vi "Perdite da a vuoto.vi"(0 "Acquisizioni vuoto":T3, 1 "Acqisizioni termica":T2) -> (15 "Perdite da prova a vuoto":T1)   [LabVIEW 2019]
uses:
  <vilib>/Analysis/NI_AALPro.lvlib
panel:
  out "XY Graph":cluster{dbl[], dbl[]}[](graph)
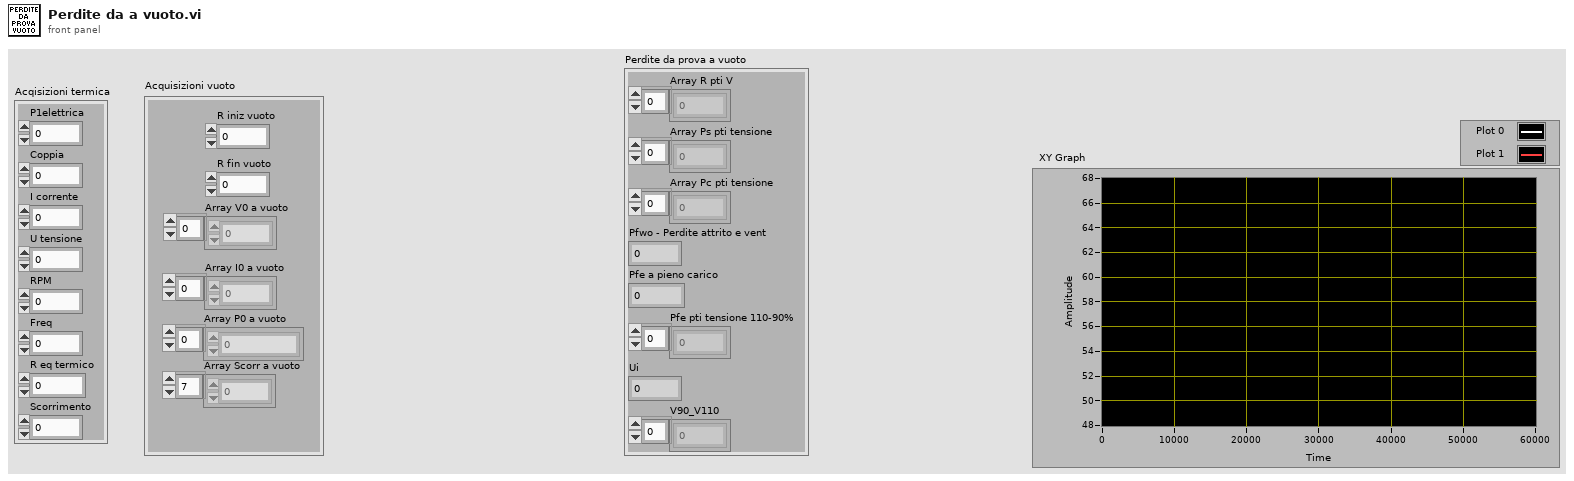
[diagram p1: front panel]
types:
  T1 = cluster{"Array R pti V":dbl[], "Array Ps pti tensione":dbl[], "Array Pc pti tensione":dbl[], "Pfwo - Perdite attrito e vent":dbl, "Pfe a pieno carico":dbl, "Pfe pti tensione 110-90% ":dbl[], "Ui":dbl, "V90_V110":dbl[]}
  T2 = cluster{"P1elettrica":dbl, "Coppia":dbl, "I corrente":dbl, "U tensione":dbl, "RPM":dbl, "Freq":dbl, "R eq termico":dbl, "Scorrimento":dbl}
  T3 = cluster{"R iniz vuoto":dbl, "R fin vuoto":dbl, "Array V0 a vuoto":dbl[], "Array I0 a vuoto":dbl[], "Array P0 a vuoto":dbl[], "Array Scorr a vuoto":dbl[]}
  T4 = cluster{"Array R pti V":dbl[], "Array Ps pti tensione":dbl[], "Array Pc pti tensione":dbl[], "Pfwo - Perdite attrito e vent":dbl, "Pfe a pieno carico":dbl, "Pfe pti tensione 110-90% ":dbl[]}
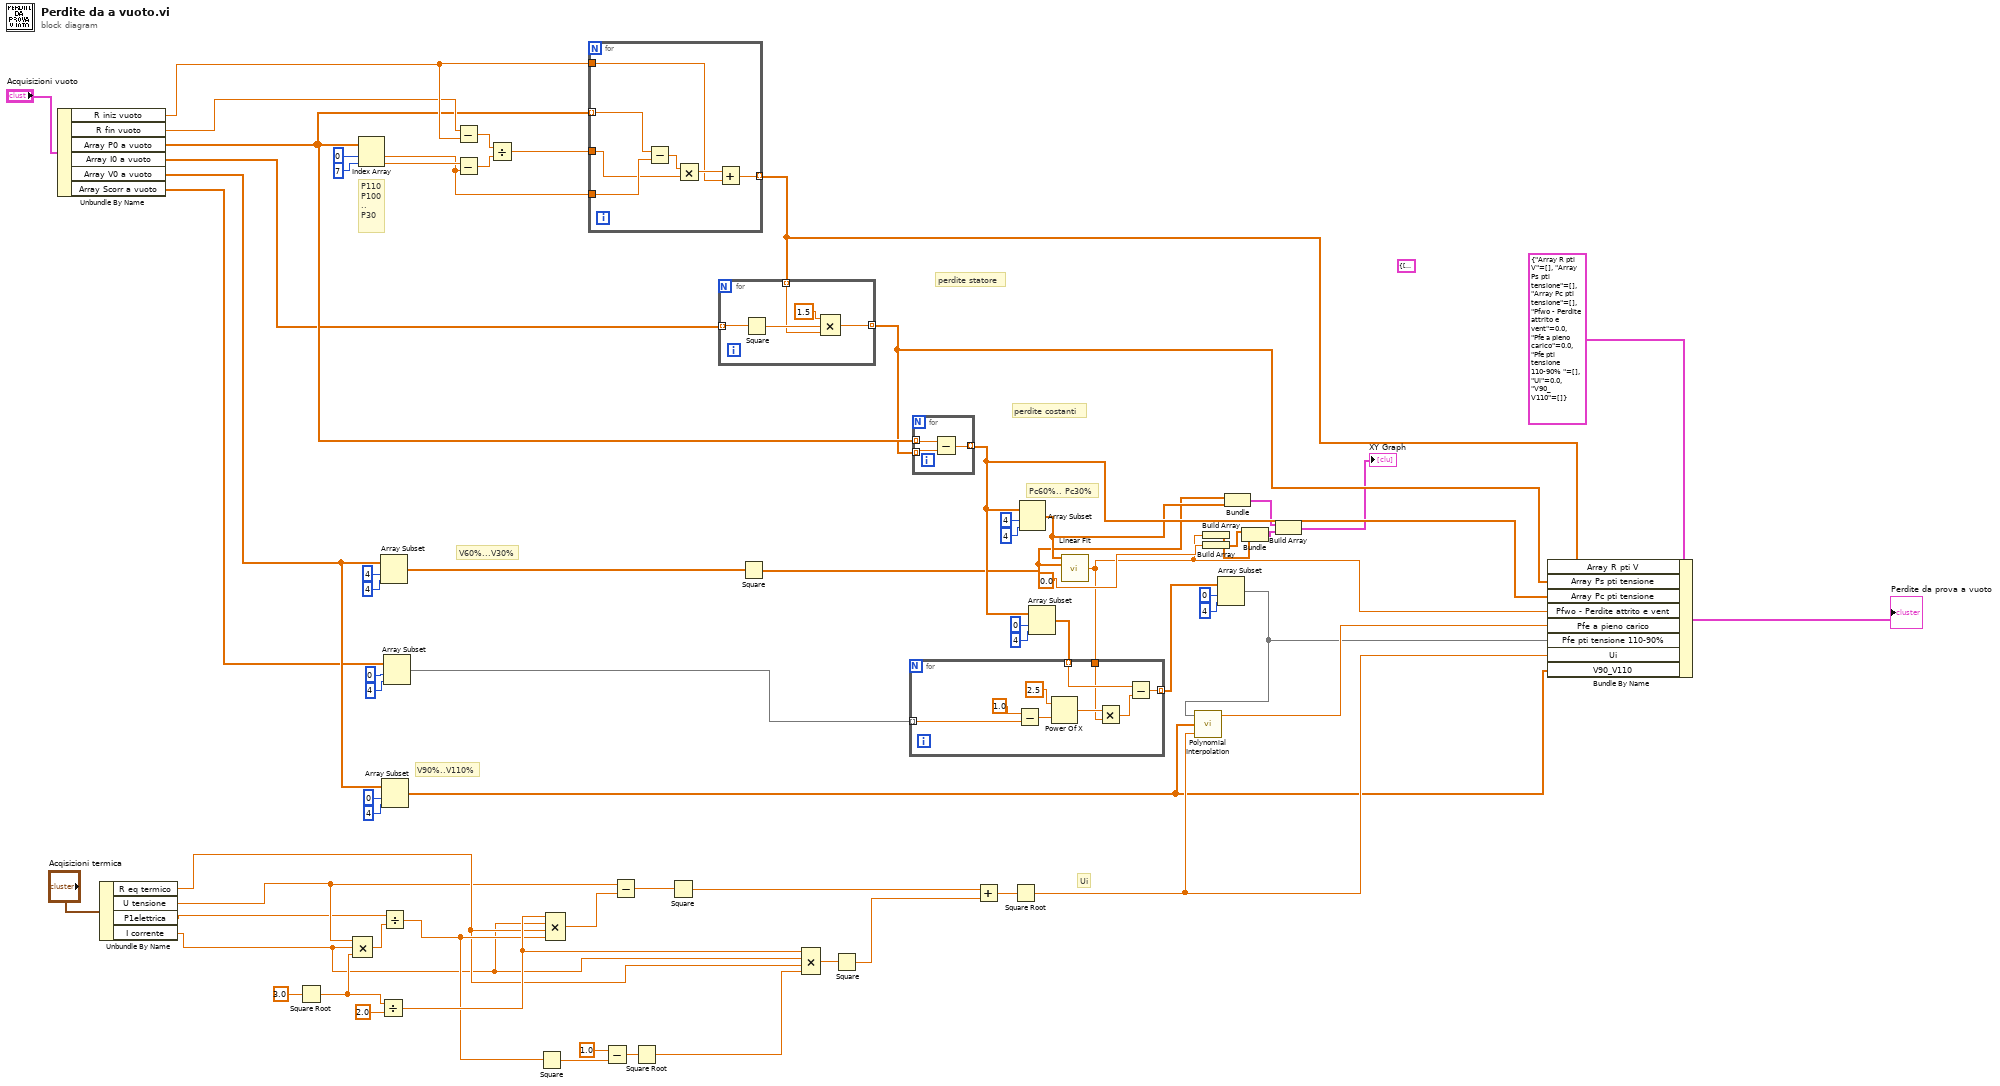
[diagram p0: block diagram]
diagram:
  (unwired) T4 {"Array R pti V"=[], "Array Ps pti tensione"=[], "Array Pc pti tensione"=[], "Pfwo - Perdite attrito e vent"=0.0, "Pfe a pieno carico"=0.0, "Pfe pti tensione 110-90% "=[]} ("Perdite da prova a vuoto")
  # "Ui"
  # "V90%..V110%"
  # "Pc60%.. Pc30%"
  # "V60%...V30%"
  # "P110\nP100\n..\nP30"
  # "perdite costanti"
  # "perdite statore"
  n1 = Unbundle By Name("Acquisizioni vuoto") -> ("R iniz vuoto"=w31:dbl, "R fin vuoto"=w30:dbl, "Array P0 a vuoto"=w29:dbl[], "Array I0 a vuoto"=w28:dbl[], "Array V0 a vuoto"=w27:dbl[], "Array Scorr a vuoto"=w24:dbl[])
  n2 = Unbundle By Name("Acqisizioni termica") -> ("R eq termico"=w36:dbl, "U tensione"=w35:dbl, "P1elettrica"=w34:dbl, "I corrente"=w33:dbl)
  n3 = Square Root(x=3.0) -> (sqrt(x)=w51:dbl)
  n4 = Compound Arithmetic op=MULTIPLY(w35, w33, w51) -> (w52:dbl)
  n5 = Index Array(array=w29, index #1=0 ("index"), index #2=7 ("index")) -> (element #1=w63:dbl, element #2=w67:dbl)
  n6 = Divide(x=w51, y=2.0) -> (x/y=w46:dbl)
  n7 = Array Subset(array=w27, index=4, length=4) -> (w13:dbl[])
  n8 = Array Subset(array=w27, index=0, length=4) -> (w2:dbl[])
  n9 = Divide(x=w34, y=w52) -> (x/y=w45:dbl)
  n10 = Array Subset(array=w24, index=0, length=4) -> (w23:dbl[])
  n11 = Subtract(x=w30, y=w31) -> (x-y=w66:dbl)
  n12 = Subtract(x=w67, y=w63) -> (x-y=w65:dbl)
  n13 = Divide(x=w66, y=w65) -> (x/y=w64:dbl)
  n14 = Square(x=w45) -> (x^2=w43:dbl)
  n15 = Compound Arithmetic op=MULTIPLY(w46, w33, w36, w45) -> (w49:dbl)
  n16 = for {
    tunnel: w29 -> [w76] mode=indexing
    tunnel: w31 -> [w71]
    tunnel: w64 -> [w73]
    tunnel: w63 -> [w75]
    tunnel: [w70] -> w22 mode=indexing
    n17 = Subtract(x=w76, y=w75) -> (x-y=w74:dbl)
    n18 = Multiply(x=w74, y=w73) -> (x*y=w72:dbl)
    n19 = Add(x=w72, y=w71) -> (x+y=w70:dbl)
  }
  n20 = Subtract(x=1.0, y=w43) -> (x-y=w42:dbl)
  n21 = Subtract(x=w35, y=w49) -> (x-y=w48:dbl)
  n22 = Square Root(x=w42) -> (sqrt(x)=w41:dbl)
  n23 = Square(x=w48) -> (x^2=w47:dbl)
  n24 = for {
    tunnel: w28 -> [w81] mode=indexing
    tunnel: w22 -> [w78] mode=indexing
    tunnel: [w77] -> w16 mode=indexing
    n25 = Square(x=w81) -> (x^2=w80:dbl)
    n26 = Compound Arithmetic op=MULTIPLY(1.5 ("value"), w80, w78) -> (w77:dbl)
  }
  n27 = Square(x=w13) -> (x^2=w4:dbl[])
  n28 = Compound Arithmetic op=MULTIPLY(w46, w33, w36, w41) -> (w40:dbl)
  n29 = Square(x=w40) -> (x^2=w39:dbl)
  n30 = for {
    tunnel: w29 -> [w84] mode=indexing
    tunnel: w16 -> [w83] mode=indexing
    tunnel: [w82] -> w17 mode=indexing
    n31 = Subtract(x=w84, y=w83) -> (x-y=w82:dbl)
  }
  n32 = Add(x=w47, y=w39) -> (x+y=w38:dbl)
  n33 = Square Root(x=w38) -> (sqrt(x)=w19:dbl)
  n34 = Array Subset(array=w17, index=4, length=4) -> (w5:dbl[])
  n35 = Array Subset(array=w17, index=0, length=4) -> (w54:dbl[])
  n36 = call <vilib>:"Linear Fit.vi"("Y"=w5, "X"=w4) -> ("intercept"=w3:dbl)  [unwired: 9 in, 4 out]
  n37 = for {
    tunnel: w54 -> [w93] mode=indexing
    tunnel: w3 -> [w86]
    tunnel: [w92] -> w12 mode=indexing
    tunnel: w23 -> [w87] mode=indexing
    n38 = Subtract(x=1.0, y=w87) -> (x-y=w89:dbl)
    n39 = Power Of X(1:w89, 2:2.5 ("y")) -> (0:w91:dbl)
    n40 = Multiply(x=w91, y=w86) -> (x*y=w85:dbl)
    n41 = Subtract(x=w93, y=w85) -> (x-y=w92:dbl)
  }
  n42 = Build Array(w3) -> (w6:dbl[])
  n43 = Build Array(0.0 ("x value")) -> (w7:dbl[])
  n44 = Array Subset(array=w12, index=0, length=4) -> (w1:dbl[])
  n45 = call <vilib>:"Polynomial Interpolation.vi"("x value"=w19, "X"=w2, "Y"=w1) -> ("interpolation value"=w21:dbl)  [unwired: 2 out]
  n46 = Bundle(w4, w5) -> (w11:cluster{dbl[], dbl[]})  [unwired: 1 in]
  n47 = Bundle(w7, w6) -> (w9:cluster{dbl[], dbl[]})  [unwired: 1 in]
  n48 = Build Array(w11, w9) -> (→"XY Graph":cluster{dbl[], dbl[]}[])
  n49 = Bundle By Name(cluster=T1 {"Array R pti V"=[], "Array Ps pti tensione"=[], "Array Pc pti tensione"=[], "Pfwo - Perdite attrito e vent"=0.0, "Pfe a pieno carico"=0.0, "Pfe pti tensione 110-90% "=[], "Ui"=0.0, "V90_V110"=[]} ("Perdite da prova a vuoto"), "Array R pti V"=w22, "Array Ps pti tensione"=w16, "Array Pc pti tensione"=w17, "Pfwo - Perdite attrito e vent"=w3, "Pfe a pieno carico"=w21, "Pfe pti tensione 110-90%"=w1, "Ui"=w19, "V90_V110"=w2) -> (→"Perdite da prova a vuoto":T1)
